vi "UDP - Transfer Groups to DSF Cluster.vi"(0 "Tx local address":string[](array[string]), 1 "Tx local port":string[](array[string]), 2 "Tx Transfer Groups":T1[](array[typedef]) {"transfers"."channels"."core"."string offset" format="%d bytes"}, 3 "Rx Transfer Groups":T1[](array[typedef]) {"transfers"."channels"."core"."string offset" format="%d bytes"}, 4 "Rx local address":string[](array[string]), 5 "Rx local port":string[](array[string])) -> (16 "DSF Cluster":T12)   [LabVIEW 2023]
uses:
  <vilib>/addons/VeriStand Custom Device Scripting APIs/Data Sharing Framework/DSF Core.lvlibp/Typedefs/DSF Engine Framework Configuration.ctl
  <vilib>/addons/VeriStand Custom Device Scripting APIs/Data Sharing Framework/DSF Core.lvlibp/Typedefs/DSF Engine Plugin Configuration.ctl
  <vilib>/addons/VeriStand Custom Device Scripting APIs/Data Sharing Framework/DSF Core.lvlibp/Typedefs/Core Plugin Configuration.ctl
  <vilib>/addons/VeriStand Custom Device Scripting APIs/Data Sharing Framework/DSF Core.lvlibp/Typedefs/DSF Timing Info.ctl
  <vilib>/addons/VeriStand Custom Device Scripting APIs/Data Sharing Framework/DSF Core.lvlibp/Typedefs/DSF Settings Info.ctl
  <vilib>/addons/VeriStand Custom Device Scripting APIs/Data Sharing Framework/DSF Core.lvlibp/Typedefs/DSF Engine Plugin Thread Configuration.ctl
  <vilib>/addons/VeriStand Custom Device Scripting APIs/Data Sharing Framework/DSF Core.lvlibp/Typedefs/Core Thread Configuration.ctl
  <vilib>/addons/VeriStand Custom Device Scripting APIs/Data Sharing Framework/DSF Core.lvlibp/Typedefs/DSF Engine Transfer Group Configuration.ctl
  <vilib>/addons/VeriStand Custom Device Scripting APIs/Data Sharing Framework/DSF Core.lvlibp/Typedefs/Core Group Configuration.ctl
  <vilib>/addons/VeriStand Custom Device Scripting APIs/Data Sharing Framework/DSF Core.lvlibp/Typedefs/DSF Direction.ctl
  <vilib>/addons/VeriStand Custom Device Scripting APIs/Data Sharing Framework/DSF Core.lvlibp/Typedefs/DSF Timeout Behavior.ctl
  <vilib>/addons/VeriStand Custom Device Scripting APIs/Data Sharing Framework/DSF Core.lvlibp/Typedefs/DSF Engine Transfer Configuration.ctl
  <vilib>/addons/VeriStand Custom Device Scripting APIs/Data Sharing Framework/DSF Core.lvlibp/Typedefs/Core Transfer Configuration.ctl
  <vilib>/addons/VeriStand Custom Device Scripting APIs/Data Sharing Framework/DSF Core.lvlibp/Typedefs/DSF Engine Channel Configuration.ctl
  <vilib>/addons/VeriStand Custom Device Scripting APIs/Data Sharing Framework/DSF Core.lvlibp/Typedefs/Core Channel Configuration.ctl
  <vilib>/addons/VeriStand Custom Device Scripting APIs/Data Sharing Framework/DSF Core.lvlibp/Typedefs/DSF Data Type.ctl
  <vilib>/addons/VeriStand Custom Device Scripting APIs/Data Sharing Framework/DSF Core.lvlibp
  <vilib>/addons/VeriStand Custom Device Scripting APIs/Data Sharing Framework/DSF Core.lvlibp/Classes/Configuration/Core/Channel/Channel Configuration.lvclass
  <vilib>/addons/VeriStand Custom Device Scripting APIs/Data Sharing Framework/DSF Core.lvlibp/Classes/Configuration/Core/Transfer/Transfer Configuration.lvclass
  <vilib>/addons/VeriStand Custom Device Scripting APIs/Data Sharing Framework/DSF Core.lvlibp/Classes/Configuration/Core/Group/Group Configuration.lvclass
  <vilib>/addons/VeriStand Custom Device Scripting APIs/Data Sharing Framework/DSF Core.lvlibp/Classes/Configuration/Core/Thread/Thread Configuration.lvclass
  <vilib>/addons/VeriStand Custom Device Scripting APIs/Data Sharing Framework/DSF Core.lvlibp/Classes/Configuration/Core/Plugin/Plugin Configuration.lvclass
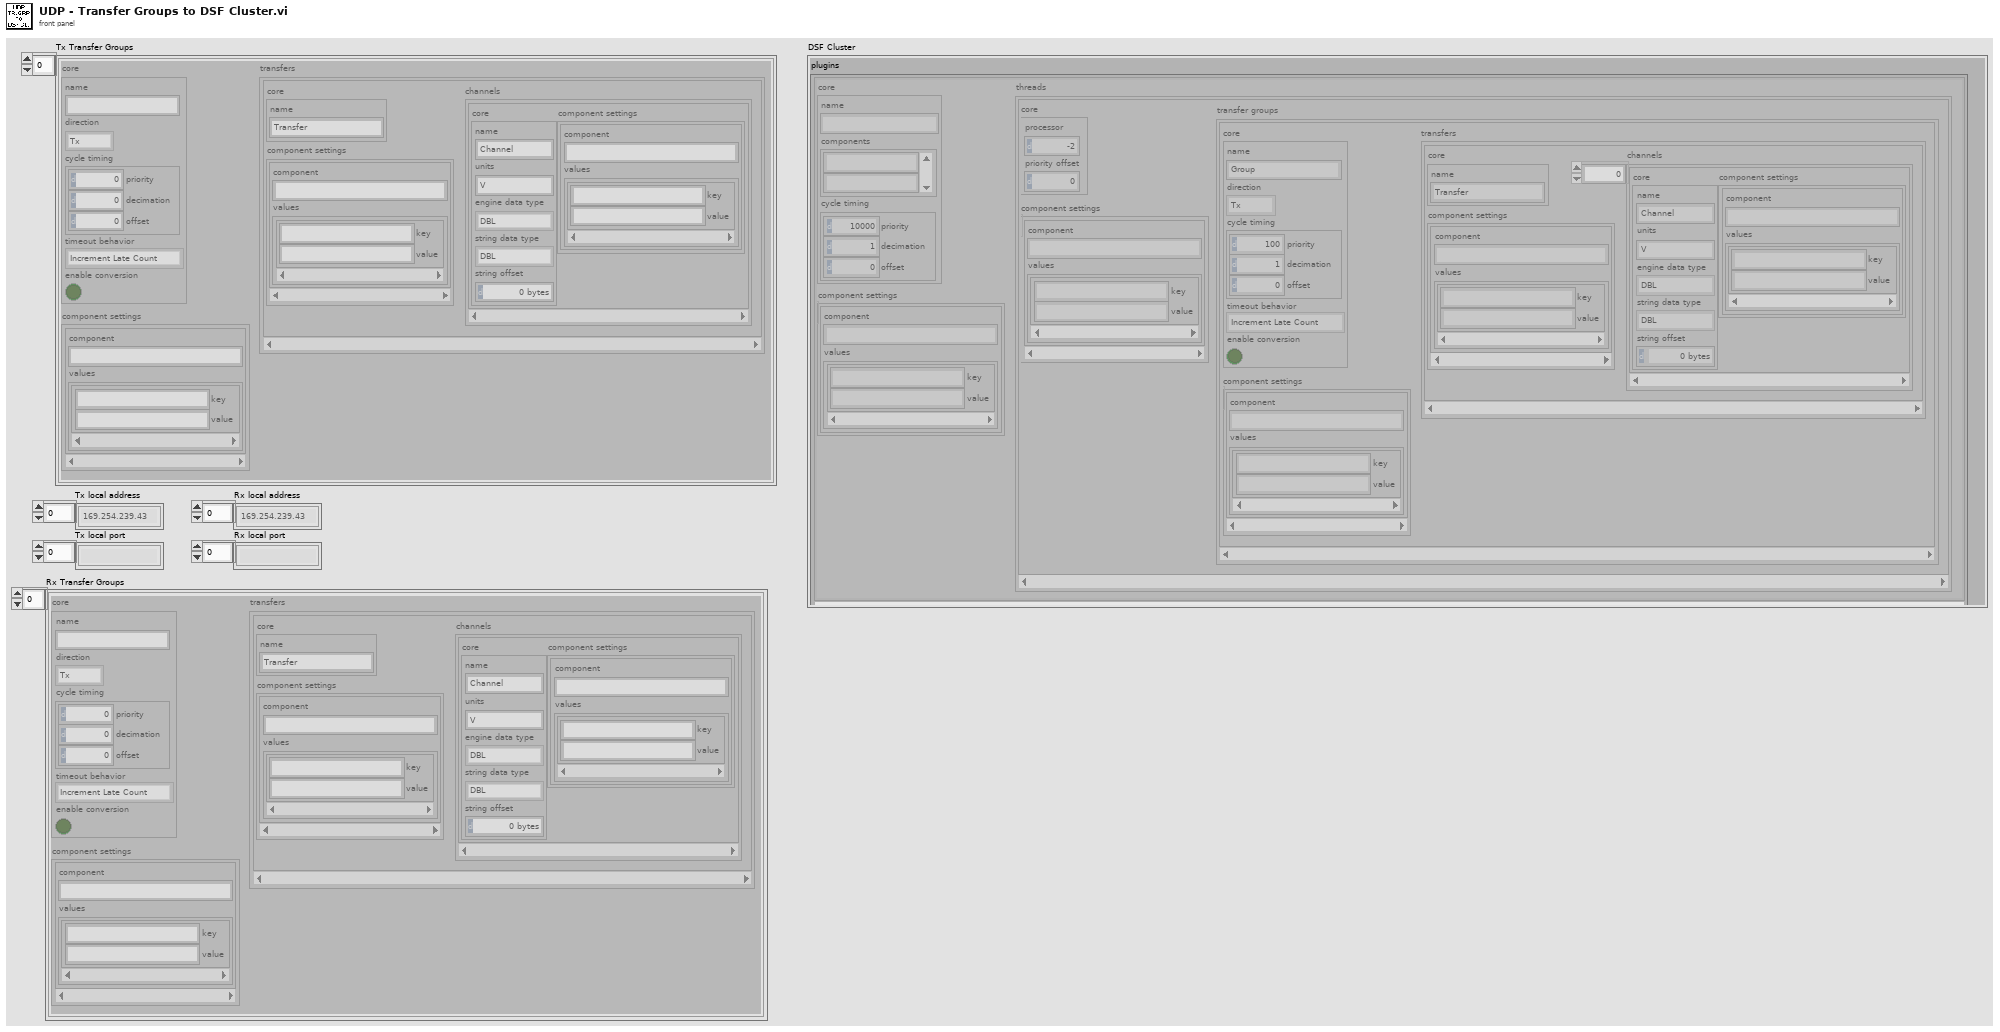
[diagram p1: front panel]
types:
  T1 = typedef "DSF Core.lvlibp/DSF Engine Transfer Group Configuration.ctl" = cluster{"core":T2, "component settings":T6[], "transfers":T7[]}
  T2 = typedef "DSF Core.lvlibp/Group Configuration.lvclass/Core Group Configuration.ctl" = cluster{"name":string, "direction":T3, "cycle timing":T4, "timeout behavior":T5, "enable conversion":bool}
  T3 = typedef "DSF Core.lvlibp/DSF Direction.ctl" = enum8{"Tx", "Rx"}
  T4 = typedef "DSF Core.lvlibp/DSF Timing Info.ctl" = cluster{"priority":u64, "decimation":u64, "offset":u64}
  T5 = typedef "DSF Core.lvlibp/DSF Timeout Behavior.ctl" = enum8{"Increment Late Count", "Throw Error"}
  T6 = typedef "DSF Core.lvlibp/DSF Settings Info.ctl" = cluster{"component":string, "values":cluster{"key":string, "value":string}[]}
  T7 = typedef "DSF Core.lvlibp/DSF Engine Transfer Configuration.ctl" = cluster{"core":T8, "component settings":T6[], "channels":T9[]}
  T8 = typedef "DSF Core.lvlibp/Transfer Configuration.lvclass/Core Transfer Configuration.ctl" = cluster{"name":string}
  T9 = typedef "DSF Core.lvlibp/DSF Engine Channel Configuration.ctl" = cluster{"core":T10, "component settings":T6[]}
  T10 = typedef "DSF Core.lvlibp/Channel Configuration.lvclass/Core Channel Configuration.ctl" = cluster{"name":string, "units":string, "engine data type":T11, "string data type":T11, "string offset":u64}
  T11 = typedef "DSF Core.lvlibp/DSF Data Type.ctl" = enum8{"Bool", "SGL", "DBL", "I8", "I16", "I32", "I64", "U8", "U16", "U32", "U64"}
  T12 = typedef "DSF Core.lvlibp/DSF Engine Framework Configuration.ctl" = cluster{"plugins":T13[]}
  T13 = typedef "DSF Core.lvlibp/DSF Engine Plugin Configuration.ctl" = cluster{"core":T14, "component settings":T6[], "threads":T15[]}
  T14 = typedef "DSF Core.lvlibp/Plugin Configuration.lvclass/Core Plugin Configuration.ctl" = cluster{"name":string, "components":string[], "cycle timing":T4}
  T15 = typedef "DSF Core.lvlibp/DSF Engine Plugin Thread Configuration.ctl" = cluster{"core":T16, "component settings":T6[], "transfer groups":T1[]}
  T16 = typedef "DSF Core.lvlibp/Thread Configuration.lvclass/Core Thread Configuration.ctl" = cluster{"processor":i32, "priority offset":i16}
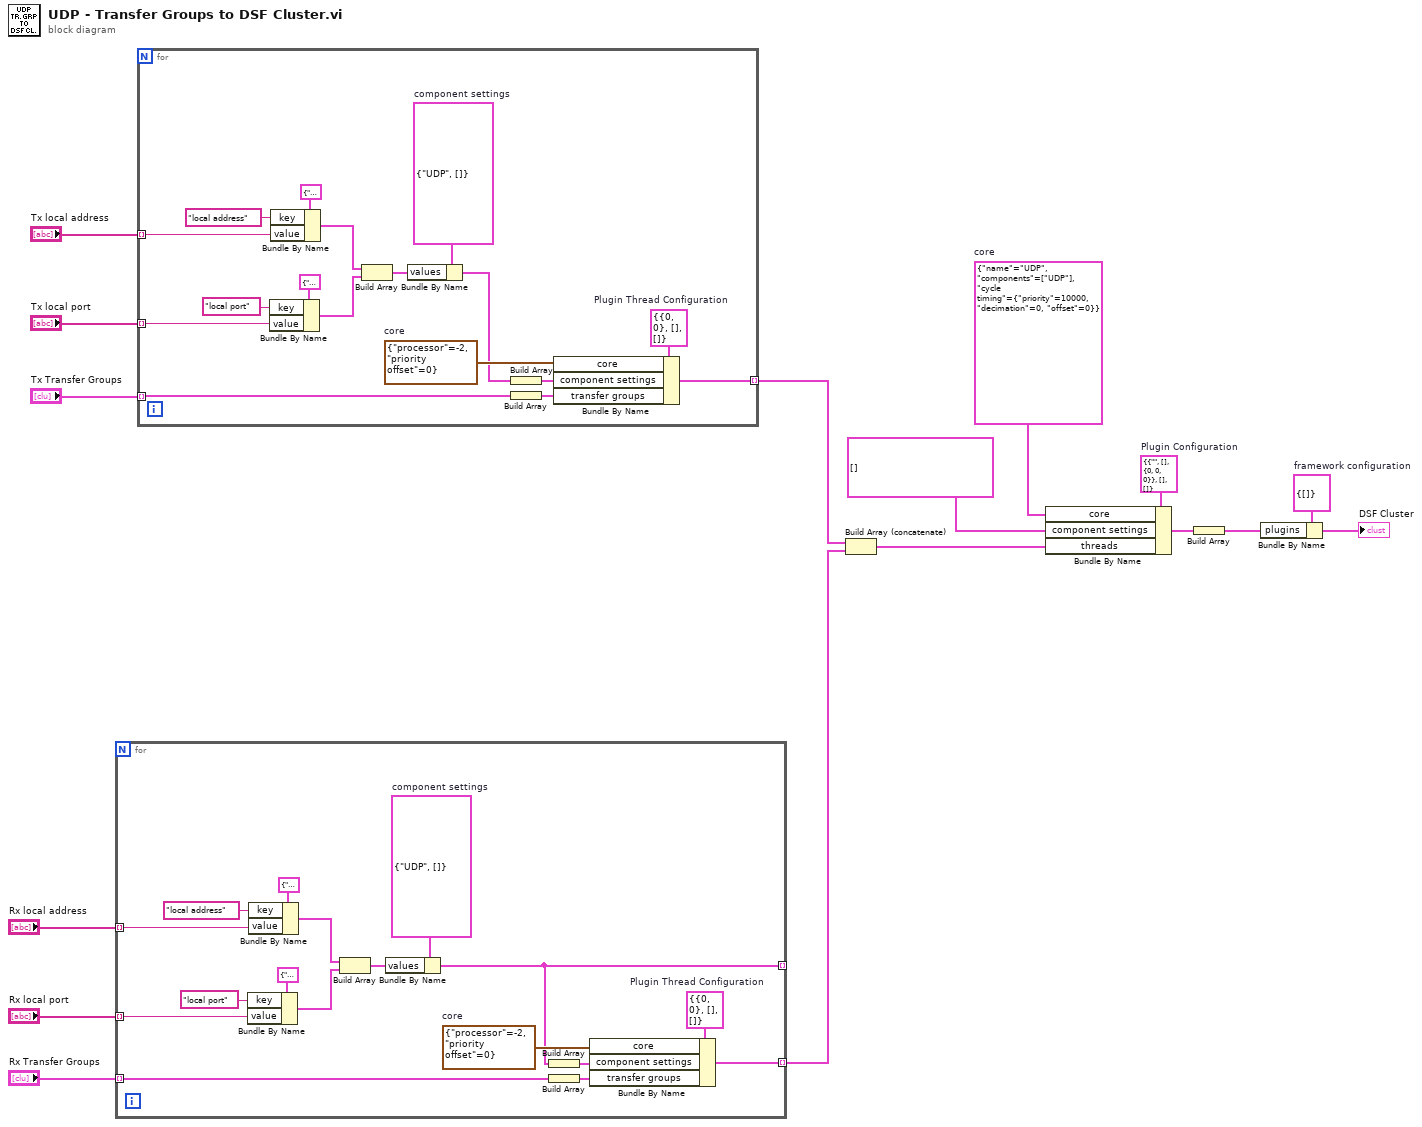
[diagram p0: block diagram]
diagram:
  w10 = T14 {"name"="UDP", "components"=["UDP"], "cycle timing"={"priority"=10000, "decimation"=0, "offset"=0}}  # core
  w13 = T13 {"core"={"name"="", "components"=[], "cycle timing"={"priority"=0, "decimation"=0, "offset"=0}}, "component settings"=[], "threads"=[]}  # Plugin Configuration
  w15 = T12 {"plugins"=[]}  # framework configuration
  n1 = for {
    tunnel: "Rx local address" -> [w31] mode=indexing
    tunnel: "Rx local port" -> [w27] mode=indexing
    tunnel: [w20] -> _ mode=indexing
    tunnel: [w21] -> w2 mode=indexing
    tunnel: "Rx Transfer Groups" -> [w17] mode=indexing
    w22 = T16 {"processor"=-2, "priority offset"=0}  # core
    w23 = T15 {"core"={"processor"=0, "priority offset"=0}, "component settings"=[], "transfer groups"=[]}  # Plugin Thread Configuration
    w25 = T6 {"component"="UDP", "values"=[]}  # component settings
    n2 = Bundle By Name(cluster=cluster{"key":string, "value":string} {"key"="", "value"=""} ("setting"), "key"="local port", "value"=w27) -> (w26:cluster{"key":string, "value":string})
    n3 = Bundle By Name(cluster=cluster{"key":string, "value":string} {"key"="", "value"=""} ("setting"), "key"="local address", "value"=w31) -> (w28:cluster{"key":string, "value":string})
    n4 = Build Array(w28, w26) -> (w24:cluster{"key":string, "value":string}[])
    n5 = Bundle By Name(cluster=w25, "values"=w24) -> (w20:T6)
    n6 = Build Array(w20) -> (w19:T6[])
    n7 = Build Array(w17) -> (w18:T1[])
    n8 = Bundle By Name(cluster=w23, "core"=w22, "component settings"=w19, "transfer groups"=w18) -> (w21:T15)
  }
  n9 = for {
    tunnel: "Tx local address" -> [w48] mode=indexing
    tunnel: "Tx local port" -> [w44] mode=indexing
    tunnel: "Tx Transfer Groups" -> [w35] mode=indexing
    tunnel: [w38] -> w3 mode=indexing
    w40 = T16 {"processor"=-2, "priority offset"=0}  # core
    w39 = T15 {"core"={"processor"=0, "priority offset"=0}, "component settings"=[], "transfer groups"=[]}  # Plugin Thread Configuration
    w42 = T6 {"component"="UDP", "values"=[]}  # component settings
    n10 = Bundle By Name(cluster=cluster{"key":string, "value":string} {"key"="", "value"=""} ("setting"), "key"="local port", "value"=w44) -> (w43:cluster{"key":string, "value":string})
    n11 = Bundle By Name(cluster=cluster{"key":string, "value":string} {"key"="", "value"=""} ("setting"), "key"="local address", "value"=w48) -> (w45:cluster{"key":string, "value":string})
    n12 = Build Array(w45, w43) -> (w41:cluster{"key":string, "value":string}[])
    n13 = Bundle By Name(cluster=w42, "values"=w41) -> (w37:T6)
    n14 = Build Array(w37) -> (w36:T6[])
    n15 = Build Array(w35) -> (w34:T1[])
    n16 = Bundle By Name(cluster=w39, "core"=w40, "component settings"=w36, "transfer groups"=w34) -> (w38:T15)
  }
  n17 = Build Array (concatenate)(w3, w2) -> (w16:T15[])
  n18 = Bundle By Name(cluster=w13, "core"=w10, "component settings"=T6[] [], "threads"=w16) -> (w12:T13)
  n19 = Build Array(w12) -> (w14:T13[])
  n20 = Bundle By Name(cluster=w15, "plugins"=w14) -> (→"DSF Cluster":T12)
